vi "LINC Format Description.vi"(1 "string in":string) -> (0 "string out":string)   [LabVIEW 2018, in "STEPkgDriver_LINC.lvlib"]
uses:
  STEPkgDriver_LINC.lvlib
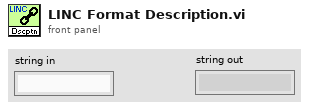
[diagram p1: front panel]
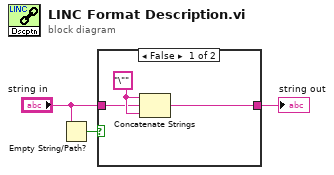
[diagram p0: block diagram]
diagram:
  n1 = Empty String/Path?(string/path="string in") -> (empty?=w1:bool)
  n2 = case shown="False" w1 {
    tunnel: "string in" -> [w5 w7]
    tunnel: [w4 w7] -> w3
    frame False {
      w6 = "\"" ("string")
      n3 = Concatenate Strings(w6, w5, w6) -> (w4:string)
    }
    frame True {
    }
  }
  "string out" <- w3
